vi "WinchPID.vi"(9 "setpoint":dbl format="%.2f", 11 "EncoderRefNum":string="My Encoder RefNum") -> (0 "Done":bool)   [LabVIEW 2014]
uses:
  <vilib>/addons/control/pid/pid.llb/PID (DBL).vi
  <vilib>/addons/control/pid/NI_PID_pid.lvlib
panel:
  out "output":dbl format="%.2f"
  in  "PID gains":T1={"proportional gain (Kc)"=1.0, "integral time (Ti, min)"=0.01, "derivative time (Td, min)"=0.0} {"derivative time (Td, min)" format="%.3f"; "integral time (Ti, min)" format="%.3f"; "proportional gain (Kc)" format="%.3f"}
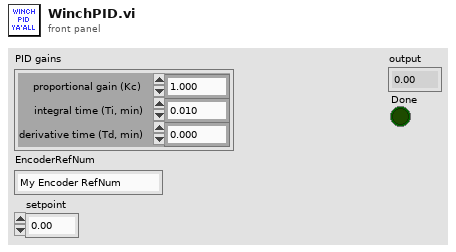
[diagram p1: front panel]
types:
  T1 = cluster{"proportional gain (Kc)":dbl, "integral time (Ti, min)":dbl, "derivative time (Td, min)":dbl}
  T2 = typedef "WPI_EncoderDevRef.ctl" = cluster{"DevStatus":errorcluster, "EncoderIndex":T3, "CounterIndex":T4, "DistancePerCount":dbl, "Decoding Type":T5}
  T3 = typedef "FPGA_EncoderIdx.ctl" = enum8{"Enc 0", "Enc 1", "Enc 2", "Enc 3", "Enc 4", "Enc 5", "Enc 6", "Enc 7", "Invalid"}
  T4 = typedef "FPGA_CounterCtrSystemIndex.ctl" = enum8{"Ctr 0", "Ctr 1", "Ctr 2", "Ctr 3", "Ctr 4", "Ctr 5", "Ctr 6", "Ctr 7", "Invalid"}
  T5 = typedef "WPI_EncoderType.ctl" = enum16{"1x", "2x", "4x"}
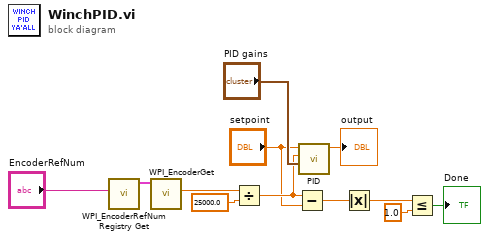
[diagram p0: block diagram]
diagram:
  n1 = call <vilib>:"WPI_EncoderRefNum Registry Get.vi"("refnum name"="EncoderRefNum") -> ("EncoderDevRef"=w10:T2)  [unwired: 9 in, 1 out]
  n2 = call <vilib>:"WPI_EncoderGet.vi"("EncoderDevRef"=w10) -> ("Distance"=w9:dbl)  [unwired: 5 in, 5 out]
  n3 = Divide(x=w9, y=25000.0) -> (x/y=w6:dbl)
  n4 = Subtract(x=w6, y="setpoint") -> (x-y=w4:dbl)
  n5 = call-poly <vilib>:"PID.vi"("PID gains"="PID gains", "process variable"=w6, "setpoint"="setpoint") -> ("output"=→"output":dbl)  [unwired: 7 in, 1 out]
  n6 = Absolute Value(x=w4) -> (abs(x)=w3:dbl)
  n7 = Less Or Equal?(x=w3, y=1.0) -> (x <= y?=→"Done":bool)
